vi "Initialize.vi"(8 "error in":errorcluster, 10 "parameters":variant, 11 "node in":refnum<class "CI Project.lvclass">) -> (0 "error out":errorcluster, 2 "summary":T2[](array[typedef]), 3 "data value reference":T1)   [LabVIEW 2014, in "CI Project.lvclass"]
doc: "Initializes the data of a node to its default state.\nThe object is not created inside of this VI, because it is created from a File depending on user selection."
uses:
  CI Project.lvclass
  <vilib>/ni/Configuration Framework/Node/Summary.ctl
  <vilib>/ni/Configuration Framework/Node/NodeRef.ctl
  <vilib>/ni/Configuration Framework/Node/NISE_CEF_Node.lvclass
  Job Initialize/Job Initialize.lvclass
  CI Project.lvclass/CI Project.ctl
  Build Job/Build Job.lvclass
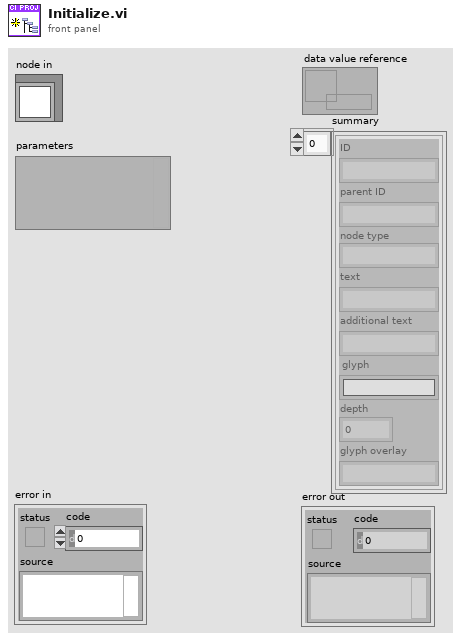
[diagram p1: front panel]
types:
  T1 = typedef "NISE_CEF_Node.lvclass/NodeRef.ctl" = refnum<data-value>
  T2 = typedef "NISE_CEF_Node.lvclass/Summary.ctl" = cluster{"ID":string, "parent ID":string, "node type":string, "text":string, "additional text":string, "glyph":string, "depth":i32, "glyph overlay":string}
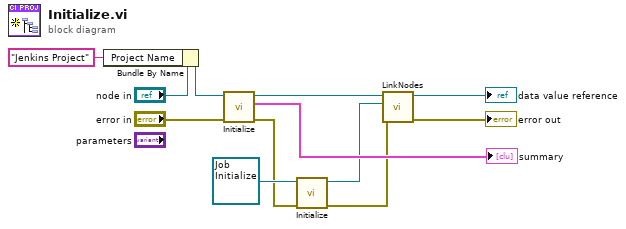
[diagram p0: block diagram]
diagram:
  n1 = Bundle By Name(cluster="node in", "Project Name"="Jenkins Project") -> (w10:refnum<class "CI Project.lvclass">)
  n2 = call-parent "Initialize.vi"("error in"="error in", "node in"=w10) -> ("error out"=w3:errorcluster, "summary"=→"summary":T2[], "data value reference"=w8:T1)  [unwired: 7 in]
  n3 = call-dynamic "Initialize.vi"("error in"=w3, "node in"=refnum<class "Job Initialize.lvclass"> refnum ("Job Initialize.lvclass")) -> ("error out"=w2:errorcluster, "data value reference"=w1:T1)  [unwired: 7 in, 1 out]
  n4 = call <vilib>:"LinkNodes.vi"("error in"=w2, "child in"=w1, "parent in"=w8) -> ("error out"=→"error out":errorcluster, "parent out"=→"data value reference":T1)  [unwired: 6 in, 1 out]
